vi "Rudyk1.vi"   [LabVIEW 2017]
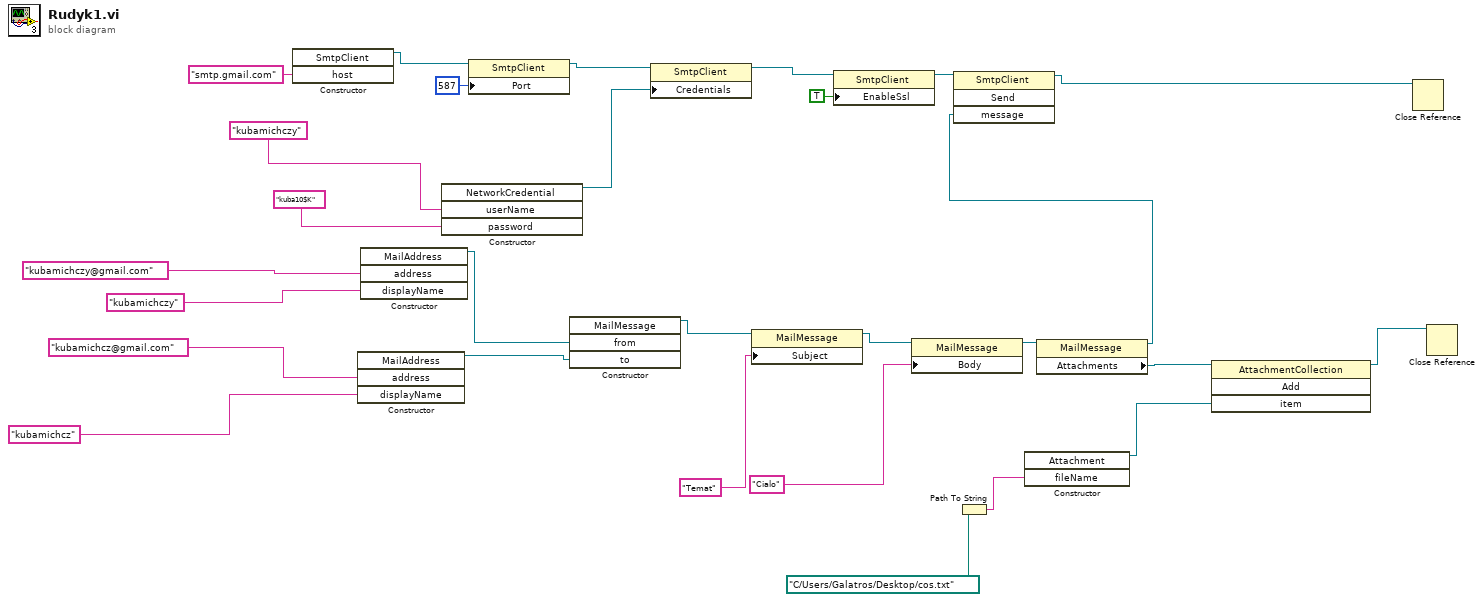
[diagram p0: block diagram]
diagram:
  n1 = constructor class="SmtpClient"("host"="smtp.gmail.com") -> (reference out=w15:refnum<k24>)  [unwired: 3 in, 3 out]
  n2 = constructor class="MailAddress"("address"="kubamichcz@gmail.com", "displayName"="kubamichcz") -> (reference out=w6:refnum<k24>)  [unwired: 3 in, 4 out]
  n3 = constructor class="MailAddress"("address"="kubamichczy@gmail.com", "displayName"="kubamichczy") -> (reference out=w5:refnum<k24>)  [unwired: 3 in, 4 out]
  n4 = constructor class="NetworkCredential"("userName"="kubamichczy", "password"="kuba10$K") -> (reference out=w20:refnum<k24>)  [unwired: 3 in, 4 out]
  n5 = property class="SmtpClient"(reference=w15, "Port"=587) -> (reference out=w19:refnum<k24>)  [unwired: 1 in, 1 out]
  n6 = constructor class="MailMessage"("from"=w5, "to"=w6) -> (reference out=w7:refnum<k24>)  [unwired: 3 in, 4 out]
  n7 = property class="SmtpClient"(reference=w19, "Credentials"=w20) -> (reference out=w21:refnum<k24>)  [unwired: 1 in, 1 out]
  n8 = property class="MailMessage"(reference=w7, "Subject"="Temat") -> (reference out=w9:refnum<k24>)  [unwired: 1 in, 1 out]
  n9 = property class="SmtpClient"(reference=w21, "EnableSsl"=TRUE) -> (reference out=w23:refnum<k24>)  [unwired: 1 in, 1 out]
  n10 = property class="MailMessage"(reference=w9, "Body"="Cialo") -> (reference out=w11:refnum<k24>)  [unwired: 1 in, 1 out]
  n11 = Path To String(path=path "C:/Users/Galatros/Desktop/cos.txt" ("Path")) -> (string=w27:string)
  n12 = constructor class="Attachment"("fileName"=w27) -> (reference out=w13:refnum<k24>)  [unwired: 3 in, 3 out]
  n13 = property class="MailMessage"(reference=w11) -> (reference out=w24:refnum<k24>, "Attachments"=w12:refnum<k24>)  [unwired: 1 in, 1 out]
  n14 = invoke class="SmtpClient" method="Send"(reference=w23, "message"=w24) -> (reference out=w26:refnum<k24>)  [unwired: 2 in, 3 out]
  n15 = invoke class="AttachmentCollection" method="Add"(reference=w12, "item"=w13) -> (reference out=w25:refnum<k24>)  [unwired: 2 in, 3 out]
  n16 = Close Reference(reference=w26) -> ()  [unwired: 1 in, 1 out]
  n17 = Close Reference(reference=w25) -> ()  [unwired: 1 in, 1 out]
